vi "TimingBar.vi"(2 "Timer Within Range":bool, 3 "Inverted":bool) -> (0 "Valve Status":bool, 1 "Color Index":i32)   [LabVIEW 2018]
panel:
  # "Outputs:\nColor Index:\n0: Normal, Off\n1: Normal, On\n2: Inverted, Off\n3: Inverted On\n\nValve State:\nReflects whether the\nvalve is on"
  # "Inputs:\nInverted: Whether or not\nthe timer treats this valve\nas \"normally open\"\n\nTimer Within Range:\nWhether or not the timer\ncurrently lies between\nthe two trigger times\nfor the valve"
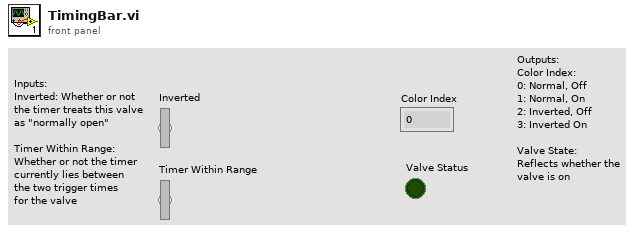
[diagram p1: front panel]
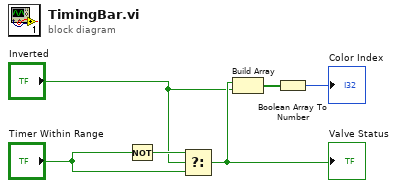
[diagram p0: block diagram]
diagram:
  n1 = Not(x="Timer Within Range") -> (.not. x?=w5:bool)
  n2 = Select(t=w5, s="Inverted", f="Timer Within Range") -> (s? t:f=w2:bool)
  "Valve Status" <- w2
  n3 = Build Array(w2, "Inverted") -> (w4:bool[])
  n4 = Boolean Array To Number(Boolean array=w4) -> (number=→"Color Index":u32)
